vi "Parallel Processing.vi"() -> ()   [LabVIEW 2023]
doc: "The Parallel Processing VI shows how to process multiple images in parallel when using a grab acquisition. The Image Manager for Grab Acquisition helper VI is used to achieve the same behavior as the driver's ring acquisition.\n\nIn this example, image processing is simulated by a time delay that can be adjusted while the VI is running. When processing is complete, Unlock the image so it can be available in the acquisition loop."
uses:
  SubVIs/Grab Manager Mode.ctl
  <vilib>/vision/driver/IMAQdx.llb/IMAQdx Buffer Number Mode.ctl
  <vilib>/vision/driver/NI_Vision_Acquisition_Software.lvlib
panel:
  out "Images Missed":u32
  in  "Processing Delay (s)":dbl(slide)=0.1 scale=0.0..1.0
  out "Images Processed":u32
  out "Current Buffer Number":u32
  in  "Processing Delay (s)":dbl(slide)=0.2 scale=0.0..1.0
  out "Images Processed":u32
  out "Current Buffer Number":u32
  in  "Number of Images":u32=30
  out "Images Behind":i32
  in  "Processing Delay (s)":dbl(slide)=0.4 scale=0.0..1.0
  out "Images Processed":u32
  out "Current Buffer Number":u32
  in  "Camera Name":refnum<k21> caption="IMAQdx Session"
  in  "Stop":bool
  # "Overview: Demonstrates how to process multiple images in parallel when using a grab acquisition.\nRequirements: Vision Acquisition Software\nInstructions:\n1. Select the Camera Name\n2. Run the VI"
  # "Worker Loop 3"
  # "Worker Loop 2"
  # "Worker Loop 1"
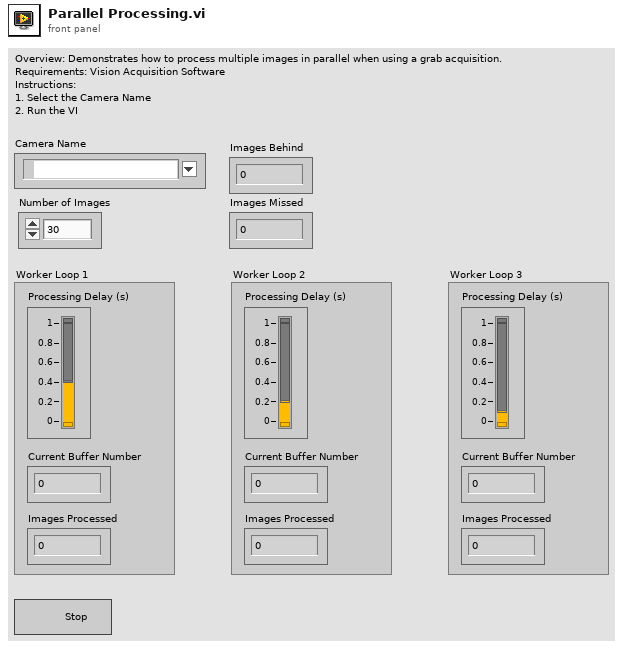
[diagram p1: front panel]
types:
  T1 = typedef "Grab Manager Mode.ctl" = enum16{"Create Processing Images", "Lock", "Add Acquired Image", "Get Acquired Image", "Unlock", "Dispose Processing Images"}
  T2 = cluster{"Number of Processing Images":u32, "Image Border Size":u32}
  T3 = typedef "IMAQdx.ctl" = refnum<k21>
  T4 = typedef "IMAQ Image.ctl" = refnum<image>
  T5 = typedef "NI_Vision_Acquisition_Software.lvlib/IMAQdx Buffer Number Mode.ctl" = enum32{"Next", "Last", "Buffer Number", "Every", "Last New"}
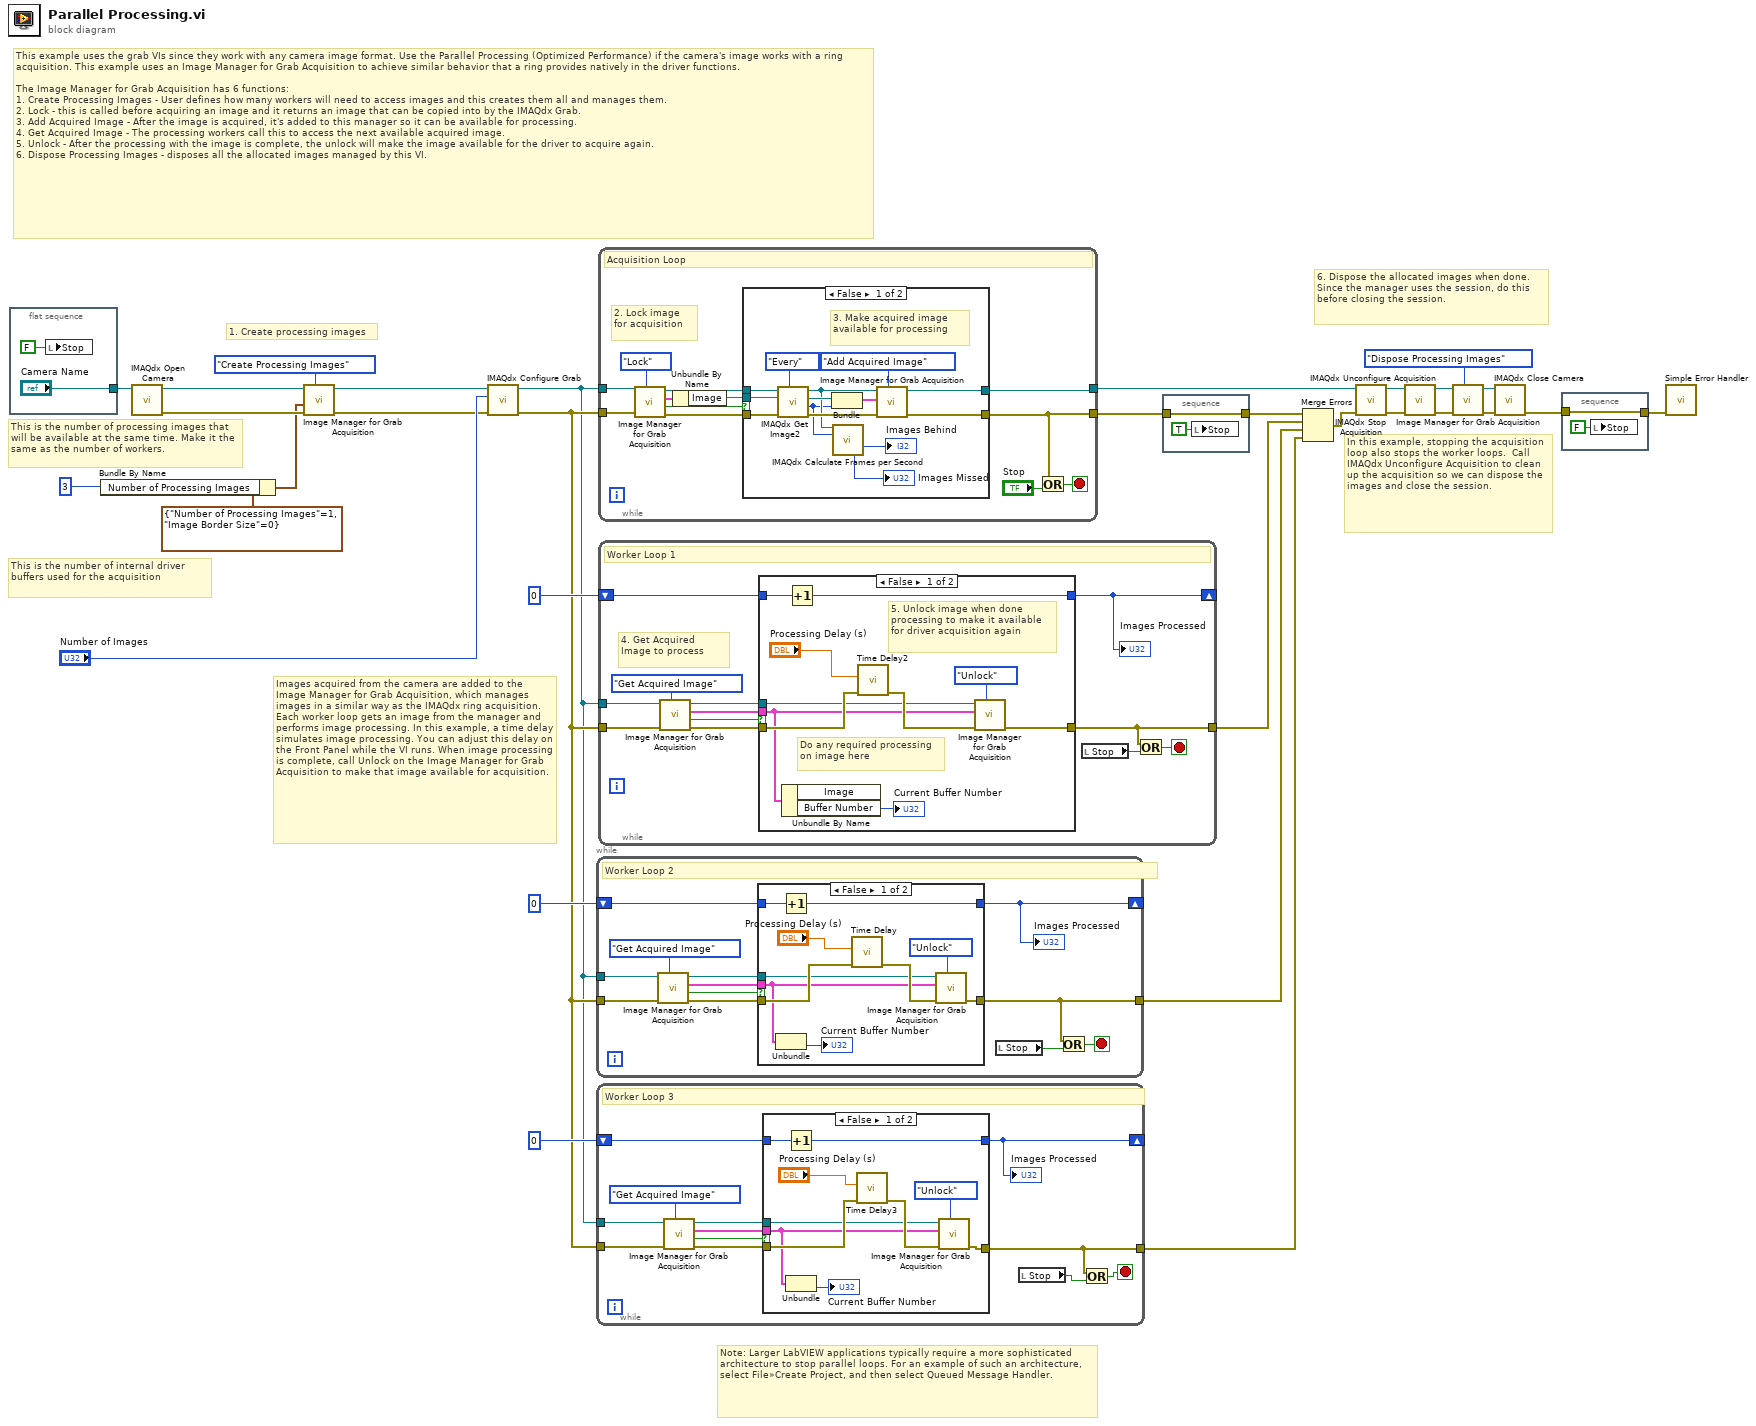
[diagram p0: block diagram]
diagram:
  # "6. Dispose the allocated images when done. Since the manager uses the session, do this before closing the session."
  # "1. Create processing images"
  # "This is the number of internal driver buffers used for the acquisition"
  # "This is the number of processing images that will be available at the same time. Make it the same as the number of workers."
  # "In this example, stopping the acquisition loop also stops the worker loops.  Call IMAQdx Unconfigure Acquisition to clean up the acquisition so we can dispose the images and close the session."
  # "Images acquired from the camera are added to the Image Manager for Grab Acquisition, which manages images in a similar way as the IMAQdx ring acquisition. Each worker loop gets an image from the manager and performs image processing. In this example, a time delay simulates image processing. You can adjust this delay on the Front Panel while the VI runs. When image processing is complete, call Unlock on the Image Manager for Grab Acquisition to make that image available for acquisition."
  # "This example uses the grab VIs since they work with any camera image format. Use the Parallel Processing (Optimized Performance) if the camera's image works with a ring acquisition. This example uses an Image Manager for Grab Acquisition to achieve similar behavior that a ring provides natively in the driver functions.\n\nThe Image Manager for Grab Acquisition has 6 functions:\n1. Create Processing Images - User defines how many workers will need to access images and this creates them all and manages them.\n2. Lock - this is called before acquiring an image and it returns an image that can be copied into by the IMAQdx Grab.\n3. Add Acquired Image - After the image is acquired, it's added to this manager so it can be available for processing.\n4. Get Acquired Image - The processing workers call this to access the next available acquired image.\n5. Unlock - After the processing with the image is complete, the unlock will make the image available for the driver to acquire again.\n6. Dispose Processing Images - disposes all the allocated images managed by this VI."
  # "Note: Larger LabVIEW applications typically require a more sophisticated architecture to stop parallel loops. For an example of such an architecture, select File»Create Project, and then select Queued Message Handler."
  n1 = flat-sequence {
    tunnel: ["Camera Name"] -> w28
    frame #0 {
      n2 = local write "Stop"(FALSE ("Stop")) -> ()
    }
  }
  n3 = Bundle By Name(cluster=T2 {"Number of Processing Images"=1, "Image Border Size"=0} ("Init Settings"), "Number of Processing Images"=u32 3 ("Number of Images")) -> (w14:T2)
  n4 = call <vilib>:"IMAQdx Open Camera.vi"("Session In"=w28) -> ("error out"=w16:errorcluster, "Session Out"=w17:T3)  [unwired: 2 in, 7 out]
  n5 = call "Image Manager for Grab Acquisition.vi"("Mode"=Grab_Manager_Mode."Create Processing Images", "error in (no error)"=w16, "Init Settings"=w14, "Session In"=w17) -> ("error out"=w10:errorcluster, "Session Out"=w13:T3)  [unwired: 4 in, 2 out]
  n6 = call <vilib>:"IMAQdx Configure Grab.vi"("error in"=w10, "Number of Buffers"="Number of Images", "Session In"=w13) -> ("error out"=w12:errorcluster, "Session Out"=w8:T3)  [unwired: 7 in]
  n7 = while {
    tunnel: [w42] -> w23
    tunnel: w8 -> [w39]
    shift-right: [w41] -> _
    shift-left: u32 0 -> [w44]
    tunnel: w12 -> [w40]
    stop <- w45 stop-if-true
    # "Worker Loop 2"
    n8 = call "Image Manager for Grab Acquisition.vi"("Mode"=Grab_Manager_Mode."Get Acquired Image", "error in (no error)"=w40, "Session In"=w39) -> ("error out"=w38:errorcluster, "No Available Image"=w37:bool, "Image Settings Out"=w34:cluster{"Image":T4, "Buffer Number":u32}, "Session Out"=w36:T3)  [unwired: 5 in]
    n9 = case shown="False" w37 {
      tunnel: [w50 w56] -> w42
      tunnel: w36 -> [w47 _]
      tunnel: w44 -> [w55 w57]
      tunnel: [w54 w57] -> w41
      tunnel: w38 -> [w52 w56]
      tunnel: w34 -> [w48 _]
      frame False {
        n10 = Unbundle(w48) -> ("Buffer Number"=→"Current Buffer Number":u32)  [unwired: 1 out]
        n11 = Increment(x=w55) -> (x+1=w54:u32)
        n12 = call "Time Delay"("error in (no error)"=w52, "Delay Time (s)"="Processing Delay (s)") -> ("error out"=w49:errorcluster)  [unwired: 9 in]
        n13 = call "Image Manager for Grab Acquisition.vi"("Mode"=Grab_Manager_Mode."Unlock", "error in (no error)"=w49, "Image Settings In"=w48, "Session In"=w47) -> ("error out"=w50:errorcluster)  [unwired: 4 in, 3 out]
      }
      frame True {
        # "Nothing to process."
      }
    }
    "Images Processed" <- w41
    n14 = local read "Stop"() -> (w43:bool)
    n15 = Or(x=w42, y=w43) -> (x .or. y?=w45:bool)
  }
  n16 = while {
    tunnel: [w66] -> w22
    tunnel: w8 -> [w64]
    shift-right: [w65] -> _
    shift-left: u32 0 -> [w68]
    tunnel: w12 -> [w62]
    stop <- w69 stop-if-true
    # "Worker Loop 3"
    n17 = call "Image Manager for Grab Acquisition.vi"("Mode"=Grab_Manager_Mode."Get Acquired Image", "error in (no error)"=w62, "Session In"=w64) -> ("error out"=w59:errorcluster, "No Available Image"=w60:bool, "Image Settings Out"=w58:cluster{"Image":T4, "Buffer Number":u32}, "Session Out"=w61:T3)  [unwired: 5 in]
    n18 = case shown="False" w60 {
      tunnel: [w75 w80] -> w66
      tunnel: w61 -> [w72 _]
      tunnel: w68 -> [w79 w81]
      tunnel: [w78 w81] -> w65
      tunnel: w59 -> [w77 w80]
      tunnel: w58 -> [w70 _]
      frame False {
        n19 = Increment(x=w79) -> (x+1=w78:u32)
        n20 = Unbundle(w70) -> ("Buffer Number"=→"Current Buffer Number":u32)  [unwired: 1 out]
        n21 = call "Time Delay3"("error in (no error)"=w77, "Delay Time (s)"="Processing Delay (s)") -> ("error out"=w74:errorcluster)  [unwired: 9 in]
        n22 = call "Image Manager for Grab Acquisition.vi"("Mode"=Grab_Manager_Mode."Unlock", "error in (no error)"=w74, "Image Settings In"=w70, "Session In"=w72) -> ("error out"=w75:errorcluster)  [unwired: 4 in, 3 out]
      }
      frame True {
        # "Empty queue or error.\nNothing to process."
      }
    }
    "Images Processed" <- w65
    n23 = local read "Stop"() -> (w67:bool)
    n24 = Or(x=w66, y=w67) -> (x .or. y?=w69:bool)
  }
  n25 = while {
    tunnel: w12 -> [w84]
    tunnel: w8 -> [w85]
    tunnel: [w82] -> w24
    tunnel: [w83] -> w21
    stop <- w92 stop-if-true
    # "2. Lock image for acquisition"
    # "Acquisition Loop"
    n26 = call "Image Manager for Grab Acquisition.vi"("Mode"=Grab_Manager_Mode."Lock", "error in (no error)"=w84, "Session In"=w85) -> ("error out"=w88:errorcluster, "No Available Image"=w89:bool, "Image Settings Out"=w87:cluster{"Image":T4, "Buffer Number":u32}, "Session Out"=w90:T3)  [unwired: 5 in]
    n27 = Unbundle By Name(w87) -> ("Image"=w86:T4)
    n28 = case shown="False" w89 {
      tunnel: [w100 w109] -> w82
      tunnel: [w99 w108] -> w83
      tunnel: w90 -> [w107 w109]
      tunnel: w88 -> [w106 w108]
      tunnel: w86 -> [w101 _]
      frame False {
        # "3. Make acquired image available for processing"
        n29 = call <vilib>:"IMAQdx Get Image2.vi"("Buffer Number Mode (Next)"=IMAQdx_Buffer_Number_Mode."Every", "error in"=w106, "Image In"=w101, "Session In"=w107) -> ("error out"=w102:errorcluster, "Buffer Number Out"=w97:u32, "Image Out"=w104:T4, "Session Out"=w98:T3)  [unwired: 4 in]
        n30 = Bundle("Image Out"=w104, "Buffer Number Out"=w97) -> (w103:cluster{"Image Out":T4, "Buffer Number Out":u32})  [unwired: 1 in]
        n31 = call <vilib>:"IMAQdx Calculate Frames per Second.vi"("Session In"=w98, "Buffer Number"=w97) -> ("Images Behind"=→"Images Behind":i32, "Images Missed"=→"Images Missed":u32)  [unwired: 7 in, 5 out]
        n32 = call "Image Manager for Grab Acquisition.vi"("Mode"=Grab_Manager_Mode."Add Acquired Image", "error in (no error)"=w102, "Image Settings In"=w103, "Session In"=w98) -> ("error out"=w99:errorcluster, "Session Out"=w100:T3)  [unwired: 4 in, 2 out]
      }
      frame True {
        # "Write to disk operation is taking longer so images aren't added back to manager. Wait until there is an available image"
      }
    }
    n33 = Or(x=w83, y="Stop") -> (x .or. y?=w92:bool)
  }
  n34 = while {
    tunnel: [w118] -> w25
    shift-right: [w117] -> _
    shift-left: u32 0 -> [w120]
    tunnel: w12 -> [w115]
    tunnel: w8 -> [w114]
    stop <- w121 stop-if-true
    # "4. Get Acquired Image to process"
    # "Worker Loop 1"
    n35 = call "Image Manager for Grab Acquisition.vi"("Mode"=Grab_Manager_Mode."Get Acquired Image", "error in (no error)"=w115, "Session In"=w114) -> ("error out"=w113:errorcluster, "No Available Image"=w112:bool, "Image Settings Out"=w111:cluster{"Image":T4, "Buffer Number":u32}, "Session Out"=w110:T3)  [unwired: 5 in]
    n36 = case shown="False" w112 {
      tunnel: w113 -> [w131 w133]
      tunnel: w111 -> [w122 _]
      tunnel: [w127 w133] -> w118
      tunnel: w120 -> [w130 w132]
      tunnel: [w129 w132] -> w117
      tunnel: w110 -> [w125 _]
      frame False {
        # "Do any required processing on image here"
        # "5. Unlock image when done processing to make it available for driver acquisition again"
        n37 = Unbundle By Name(w122) -> ("Buffer Number"=→"Current Buffer Number":u32)  [unwired: 1 out]
        n38 = Increment(x=w130) -> (x+1=w129:u32)
        n39 = call "Time Delay2"("error in (no error)"=w131, "Delay Time (s)"="Processing Delay (s)") -> ("error out"=w126:errorcluster)  [unwired: 9 in]
        n40 = call "Image Manager for Grab Acquisition.vi"("Mode"=Grab_Manager_Mode."Unlock", "error in (no error)"=w126, "Image Settings In"=w122, "Session In"=w125) -> ("error out"=w127:errorcluster)  [unwired: 4 in, 3 out]
      }
      frame True {
        # "Nothing to process."
      }
    }
    "Images Processed" <- w117
    n41 = local read "Stop"() -> (w119:bool)
    n42 = Or(x=w118, y=w119) -> (x .or. y?=w121:bool)
  }
  n43 = stacked-sequence {
    tunnel: [w134] -> w20
    tunnel: w21 -> [w134]
    frame #0 {
      n44 = local write "Stop"(TRUE ("Stop")) -> ()
    }
  }
  n45 = Merge Errors(w20, w25, w23, w22) -> (w6:errorcluster)
  n46 = call <vilib>:"IMAQdx Stop Acquisition.vi"("error in"=w6, "Session In"=w24) -> ("error out"=w26:errorcluster, "Session Out"=w27:T3)  [unwired: 8 out]
  n47 = call <vilib>:"IMAQdx Unconfigure Acquisition.vi"("error in"=w26, "Session In"=w27) -> ("error out"=w5:errorcluster, "Session Out"=w4:T3)  [unwired: 8 out]
  n48 = call "Image Manager for Grab Acquisition.vi"("Mode"=Grab_Manager_Mode."Dispose Processing Images", "error in (no error)"=w5, "Session In"=w4) -> ("error out"=w2:errorcluster, "Session Out"=w3:T3)  [unwired: 5 in, 2 out]
  n49 = call <vilib>:"IMAQdx Close Camera.vi"("error in"=w2, "Session In"=w3) -> ("error out"=w1:errorcluster)  [unwired: 9 out]
  n50 = stacked-sequence {
    tunnel: [w136] -> w19
    tunnel: w1 -> [w136]
    frame #0 {
      n51 = local write "Stop"(FALSE ("Stop")) -> ()
    }
  }
  n52 = call <vilib>:"Simple Error Handler.vi"("error in (no error)"=w19) -> ()  [unwired: 4 in, 5 out]
